vi "ExDataFileToSpreadsheet.vi"() -> ()   [LabVIEW 2010]
uses:
  <vilib>/Utility/file.llb/Write To Spreadsheet File (DBL).vi
panel:
  in  "Input File Name":path
  in  "Spreadsheet File Name (include .xls extension)":path
  in  "Input File Operation":u32=6
  in  "Input FileType":u32=67371008
  out "error out":errorcluster
  in  "error in (no error)":errorcluster
  # "ExDataFileToSpreadsheet.vi\nThis VI will open the input file and save it to the\noutput file.  Note that the full path names\nmust be provided for both input and output files."
  # "TIF   = 67174400\n  SPE = 67371008\n  PMI  = 67436544"
  # "6 = Read Only"
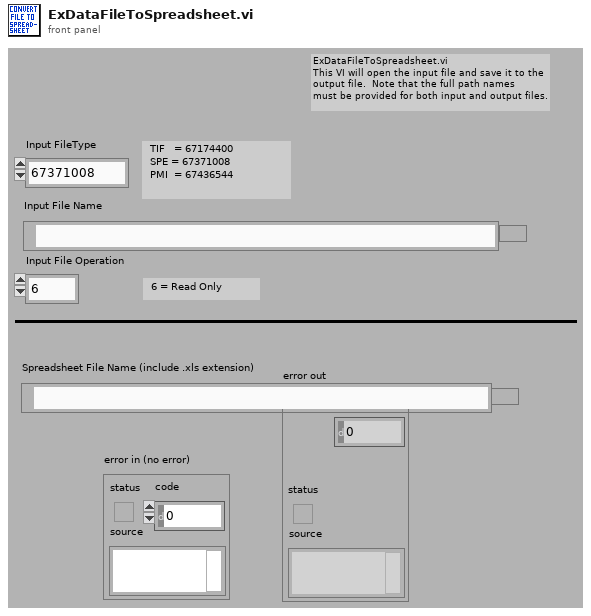
[diagram p1: front panel]
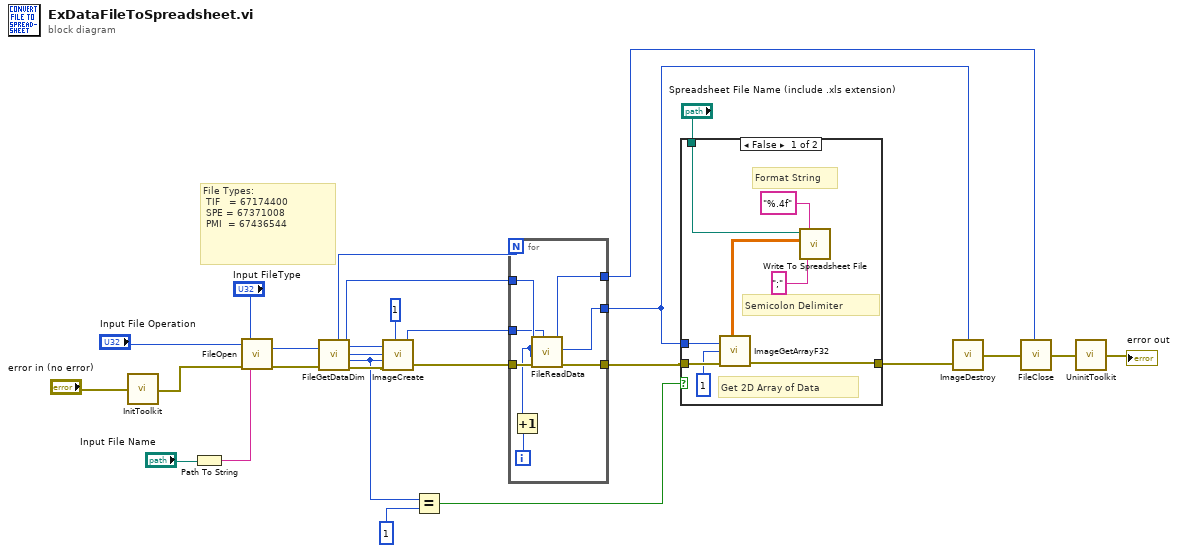
[diagram p0: block diagram]
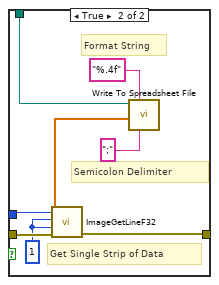
[diagram p2: hidden frame]
diagram:
  # "File Types:\n TIF   = 67174400\n SPE = 67371008\n PMI  = 67436544"
  n1 = call <userlib>:"InitToolkit.vi"("error in"="error in (no error)") -> ("error out"=w13:errorcluster)
  n2 = Path To String(path="Input File Name") -> (string=w4:string)
  n3 = call <userlib>:"FileOpen.vi"("error in"=w13, "File Operations"="Input File Operation", "FileName"=w4, "File Type"="Input FileType") -> ("error out"=w25:errorcluster, "File Handle"=w24:u32)
  n4 = call <userlib>:"FileGetDataDim.vi"("File Handle"=w24, "error in"=w25) -> ("Number of Frames"=w22:u32, "Data Type"=w6:u32, "File Handle"=w20:u32, "X dim"=w8:u32, "Y dim"=w5:u32, "error out"=w23:errorcluster)
  n5 = call <userlib>:"ImageCreate.vi"("X dimension"=w8, "Y dimension"=w5, "Data Type"=w6, "error in"=w23, "Number Of Frames"=1) -> ("Image Handle"=w19:u32, "error out"=w3:errorcluster)
  n6 = Equal?(x=w6, y=1) -> (x = y?=w11:bool)
  n7 = for {
    N: w22 -> [_]
    tunnel: w3 -> [w35]
    tunnel: w20 -> [w34]
    tunnel: w19 -> [w33]
    tunnel: [w28] -> w2
    tunnel: [w30] -> w18
    tunnel: [w29] -> w7
    i -> [w32]
    n8 = Increment(x=w32) -> (x+1=w31:i32)
    n9 = call <userlib>:"FileReadData.vi"("File Handle"=w34, "Start Frame"=w31, "End Frame"=w31, "error in"=w35, "Image Handle"=w33) -> ("File Handle"=w30:u32, "Image Handle"=w29:u32, "error out"=w28:errorcluster)
  }
  n10 = case shown="False" w11 {
    tunnel: w2 -> [w40 w50]
    tunnel: [w37 w51] -> w1
    tunnel: w7 -> [w36 w49]
    tunnel: "Spreadsheet File Name (include .xls extension)" -> [w41 w44]
    frame False {
      # "Semicolon Delimiter"
      # "Format String"
      # "Get 2D Array of Data"
      n11 = call <userlib>:"ImageGetArrayF32.vi"("error in"=w40, "Z position"=1, "Image Handle"=w36) -> ("error out"=w37:errorcluster, "Array Float 32"=w38:sgl[][])  [unwired: 1 out]
      n12 = call-poly <vilib>:"Write To Spreadsheet File.vi"("delimiter (\\t)"=";", "format (%.3f)"="%.4f", "2D data"=w38, "file path (dialog if empty)"=w41) -> ()  [unwired: 4 in, 1 out]
    }
    frame True {
      w48 = 1
      # "Semicolon Delimiter"
      # "Format String"
      # "Get Single Strip of Data"
      n13 = call <userlib>:"ImageGetLineF32.vi"("error in"=w50, "Z Position"=w48, "Y Position"=w48, "Data Handle"=w49) -> ("error out"=w51:errorcluster, "Array F32"=w45:sgl[])  [unwired: 1 out]
      n14 = call-poly <vilib>:"Write To Spreadsheet File.vi"("delimiter (\\t)"=";", "format (%.3f)"="%.4f", "1D data"=w45, "file path (dialog if empty)"=w44) -> ()  [unwired: 4 in, 1 out]
    }
  }
  n15 = call <userlib>:"ImageDestroy.vi"("error in"=w1, "Data handle"=w7) -> ("error out"=w17:errorcluster)
  n16 = call <userlib>:"FileClose.vi"("error in"=w17, "File Handle"=w18) -> ("error out"=w15:errorcluster)
  n17 = call <userlib>:"UninitToolkit.vi"("error in"=w15) -> ("error out"=→"error out":errorcluster)
